vi "Tosca-Get Message Queue.vi"() -> (4 "Message Queue":refnum<queue>, 15 "error out":errorcluster)   [LabVIEW 2020]
uses:
  Tosca-Message.ctl
  Tosca-Message Action.ctl
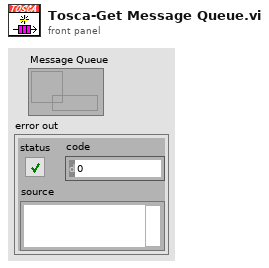
[diagram p1: front panel]
types:
  T1 = typedef "Tosca-Message.ctl" = cluster{"Action":T2, "Time":u32, "State":i32, "Events":bool[], "Error":errorcluster}
  T2 = typedef "Tosca-Message Action.ctl" = enum16{"None", "Update", "Events", "Timeout", "Error", "Abort"}
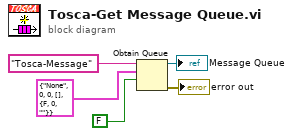
[diagram p0: block diagram]
diagram:
  n1 = Obtain Queue(name (unnamed)="Tosca-Message", element data type=T1 {"Action"=enum."None", "Time"=0, "State"=0, "Events"=[], "Error"={"status"=FALSE, "code"=0, "source"=""}} ("Data"), create if not found? (T)=FALSE) -> (queue out=→"Message Queue":refnum<queue>, error out=→"error out":errorcluster)  [unwired: 2 in, 1 out]
